vi "G#Debugger_SetCachedRef.vi"(0 "MethodVIref":refnum<vi>, 5 "error in (no error)":errorcluster) -> (19 "error out":errorcluster)   [LabVIEW 2020, in "G#Debugger.lvlib"]
doc: "Sets the cached reference to the VI to be executed."
uses:
  G#Debugger.lvlib
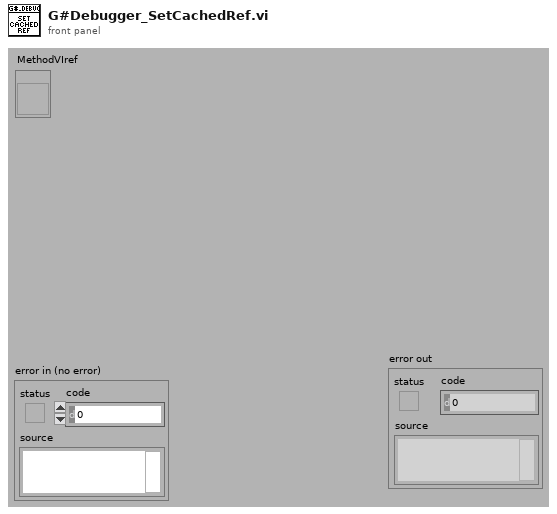
[diagram p1: front panel]
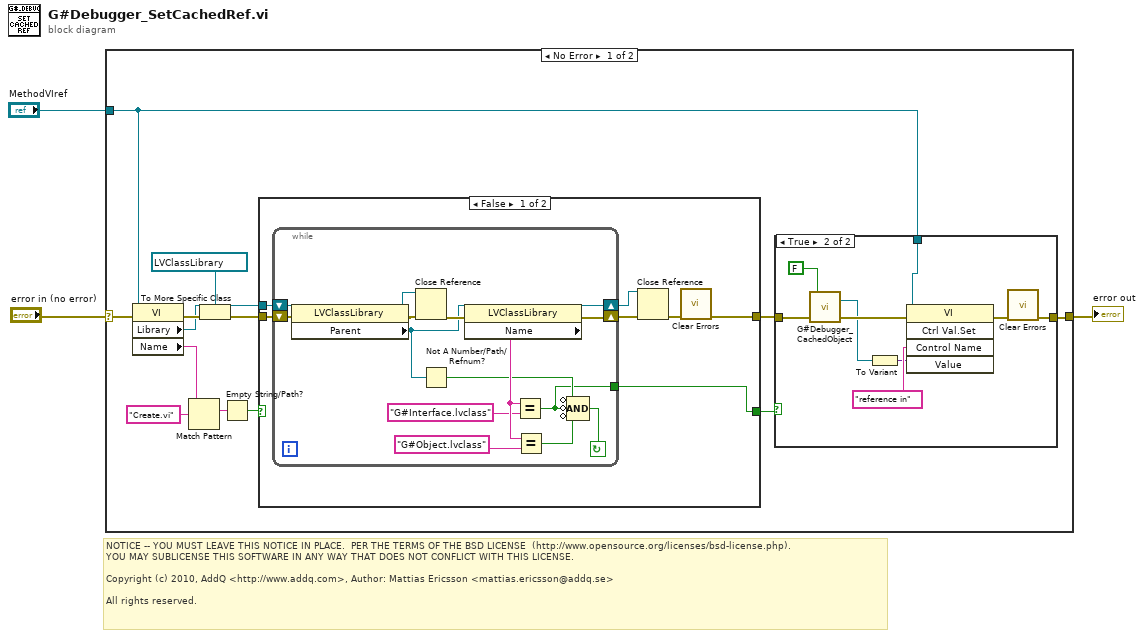
[diagram p0: block diagram]
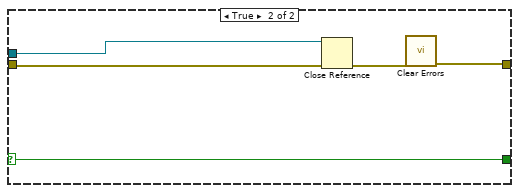
[diagram p2: hidden frame]
diagram:
  # "NOTICE -- YOU MUST LEAVE THIS NOTICE IN PLACE.  PER THE TERMS OF THE BSD LICENSE  (http://www.opensource.org/licenses/bsd-license.php).\nYOU MAY SUBLICENSE THIS SOFTWARE IN ANY WAY THAT DOES NOT CONFLICT WITH THIS LICENSE.\n\nCopyright (c) 2010, AddQ <http://www.addq.com>, Author: Mattias Ericsson <mattias.ericsson@addq.se>\n\nAll rights reserved."
  n1 = case shown="No Error" "error in (no error)" {
    selector: "error in (no error)" -> [w17 w55]
    tunnel: [w14 w55] -> w2
    tunnel: "MethodVIref" -> [w13 _]
    frame No Error {
      n2 = property class="VI"(reference=w13, error in=w17) -> (error out=w11:errorcluster, "Library"=w8:refnum<vi>, "Name"=w12:string)  [unwired: 1 out]
      n3 = Match Pattern(string=w12, regular expression="Create.vi") -> (match substring=w16:string)  [unwired: 1 in, 3 out]
      n4 = To More Specific Class(target class=refnum<vi> refnum ("reference"), reference=w8, error in=w11) -> (specific class reference=w7:refnum<vi>, error out=w10:errorcluster)
      n5 = Empty String/Path?(string/path=w16) -> (empty?=w6:bool)
      n6 = case shown="False" w6 {
        selector: w6 -> [_ w44]
        tunnel: w10 -> [w24 w41]
        tunnel: w7 -> [w23 w40]
        tunnel: [w22 w44] -> w5
        tunnel: [w18 w43] -> w4
        frame False {
          n7 = while {
            shift-right: [w27] -> w20
            shift-left: w23 -> [w38]
            tunnel: [w28] -> w22
            shift-right: [w25] -> w21
            shift-left: w24 -> [w39]
            stop <- w26 continue-if-true
            n8 = property class="LVClassLibrary"(reference=w38, error in=w39) -> (reference out=w36:refnum<vi>, error out=w37:errorcluster, "Parent"=w30:refnum<vi>)
            n9 = Close Reference(reference=w36, error in (no error)=w37) -> (error out=w31:errorcluster)
            n10 = Not A Number/Path/Refnum?(number/path/refnum=w30) -> (NaN/Path/Refnum?=w29:bool)
            n11 = property class="LVClassLibrary"(reference=w30, error in=w31) -> (reference out=w27:refnum<vi>, error out=w25:errorcluster, "Name"=w35:string)
            n12 = Equal?(x=w35, y="G#Interface.lvclass") -> (x = y?=w28:bool)
            n13 = Equal?(x=w35, y="G#Object.lvclass") -> (x = y?=w32:bool)
            n14 = Compound Arithmetic op=AND(invert w29, invert w28, invert w32) -> (w26:bool)
          }
          n15 = Close Reference(reference=w20, error in (no error)=w21) -> (error out=w19:errorcluster)
          n16 = call <vilib>:"Clear Errors.vi"("error in (no error)"=w19) -> ("error out"=w18:errorcluster)  [unwired: 5 in, 1 out]
        }
        frame True {
          n17 = Close Reference(reference=w40, error in (no error)=w41) -> (error out=w42:errorcluster)
          n18 = call <vilib>:"Clear Errors.vi"("error in (no error)"=w42) -> ("error out"=w43:errorcluster)  [unwired: 5 in, 1 out]
        }
      }
      n19 = case shown="True" w5 {
        tunnel: w4 -> [w45 w50]
        tunnel: [w45 w52] -> w14
        tunnel: w13 -> [_ w51]
        frame False {
          # "Constructor -> Don't set ref!"
        }
        frame True {
          n20 = call "G#Debugger_CachedObject.vi"("error in (no error)"=w50, "set"=FALSE) -> ("cached object out"=w46:refnum<class "G#Object.lvclass">, "error out"=w49:errorcluster)  [unwired: 15 in, 1 out]
          n21 = To Variant(anything=w46) -> (Variant=w47:variant)
          n22 = invoke class="VI" method="Ctrl Val.Set"(reference=w51, error in=w49, "Control Name"="reference in", "Value"=w47) -> (error out=w53:errorcluster)  [unwired: 1 in, 4 out]
          n23 = call <vilib>:"Clear Errors.vi"("error in (no error)"=w53) -> ("error out"=w52:errorcluster)  [unwired: 5 in, 1 out]
        }
      }
    }
    frame Error {
    }
  }
  "error out" <- w2
